vi "Main.vi"(10 "Sub Panel":refnum<vi>, 11 "Module Admin":refnum<class "Delacor_lib_QMH_Module Admin.lvclass">) -> ()   [LabVIEW 2019, in "Save DB_SQLite.lvlib"]
doc: "This template is based off of the Queued Message Handler design pattern and the Queued Message Handler project template that ships with LabVIEW.\n\nThe main difference is that the queue is private to this module and communication between modules is performed via Broadcast and Request events.\n\nRequest events are wrapped in public API methods and are handled in the Event Handling Loop (EHL) of this VI. Any module can register for Broadcast events sent by this module. The EHL generates messages based on user interface actions.\n\nThe Message Handling Loop (MHL) processes messages generated by the EHL, or by other messages. The messages are string values, so new messages can be added easily to the Message Cases case structure in the MHL. Each message cluster can also provide an optional value for Message Data, which is a variant that can be converted to whatever message-specific data is required.\n_____\nBased on Delacor QMH Project Template 5.0.0.82."
uses:
  Save DB_SQLite.lvlib
  <vilib>/Delacor/Delacor QMH/Libraries/Module Admin_class/Delacor_lib_QMH_Module Admin.lvclass
  Module Data--cluster.ctl
  Stop helper loop Argument--cluster.ctl
  Stop Argument--cluster.ctl
  <vilib>/Delacor/Delacor QMH/Libraries/Message Queue_class/Delacor_lib_QMH_Message Queue.lvclass/Delacor_lib_QMH_Message Queue.ctl
  <vilib>/Delacor/Delacor QMH/Libraries/Module Admin_class/Delacor_lib_QMH_Module Admin.lvclass/Delacor_lib_QMH_Module Admin.ctl
  <vilib>/Utility/miscctls.llb/LVPointTypeDef.ctl
  <vilib>/drjdpowell/SQLite Library/SQL Connection/Open (path).vi
  <vilib>/Delacor/Delacor QMH/Libraries/Message Queue_class/Delacor_lib_QMH_Enqueue Message (Single).vi
  <vilib>/Delacor/Delacor QMH/Libraries/Module Admin_class/Delacor_lib_QMH_Get External Launch.vi
  <vilib>/drjdpowell/SQLite Library/SQL Connection/Open (string).vi
  <vilib>/AdvancedString/Path To Command Line String.vi
  <vilib>/drjdpowell/SQLite Library/SQL Connection/Execute SQL (No results).vi
  <vilib>/Utility/error.llb/Error Cluster From Error Code.vi
  <vilib>/drjdpowell/SQLite Library/SQL Connection/Connection.lvclass
  <vilib>/ErrorRing/Error Ring.xnode
  <vilib>/Delacor/Delacor QMH/Libraries/Message Queue_class/Delacor_lib_QMH_Message Queue.lvclass
  <vilib>/drjdpowell/SQLite Library/SQLite.lvlib
  Analisis/Analisis.lvlib
panel:
  out "error out":errorcluster
  out "Status":string
types:
  T1 = typedef "Save DB_SQLite.lvlib/Request Events--cluster.ctl" = cluster{"Stop Module":refnum<user-event>, "Show Panel":refnum<user-event>, "Hide Panel":refnum<user-event>, "Get Module Execution Status":refnum<user-event>, "Show Diagram":refnum<user-event>, "Start Helper Loop":refnum<user-event>, "Stop helper loop":refnum<user-event>, "Set Waveform":refnum<user-event>, "Save_Data_From_Analisis":refnum<user-event>}
  T2 = typedef "Save DB_SQLite.lvlib/Module Data--cluster.ctl" = cluster{"Status":string}
  T3 = typedef "Save DB_SQLite.lvlib/Stop helper loop Argument--cluster.ctl" = cluster{"Boolean":bool}
  T4 = enum32{"invalid lock state", "Not Locked", "Locked (No Password)", "Password-protected"}
  T5 = typedef "Save DB_SQLite.lvlib/Stop Argument--cluster.ctl" = cluster{"Origin":string, "Exit via Stop Module Req?":bool, "Wait for Module to stop?":bool}
  T6 = typedef "LVPointTypeDef.ctl" = cluster{"Horizontal":i16, "Vertical":i16}
  T7 = enum32{"Invalid", "Standard", "Closed", "Hidden", "Minimized", "Maximized"}
  T8 = cluster{"Humedad":dbl, "Temperatura":dbl, "Voltaje":dbl, "Corriente":dbl, "Resistencia":i32}
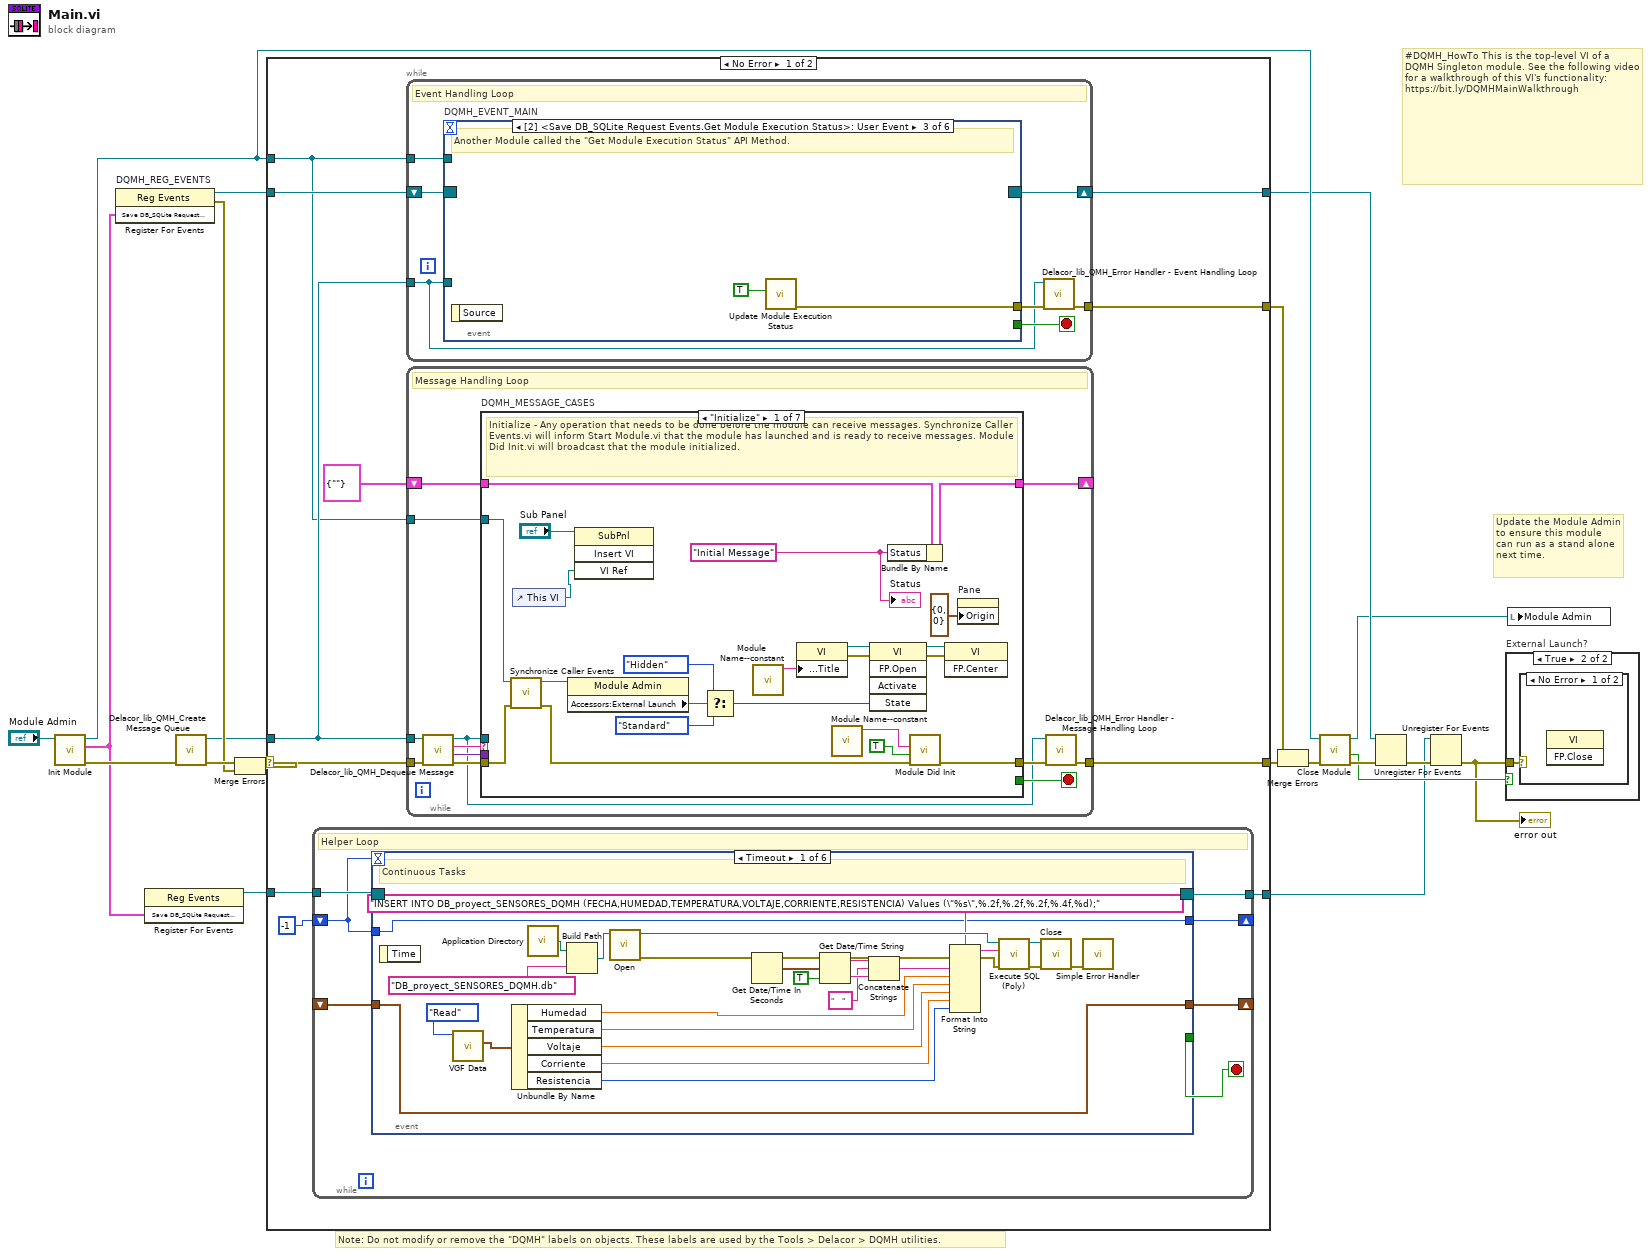
[diagram p0: block diagram]
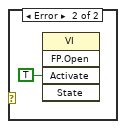
[diagram p3: hidden frame]
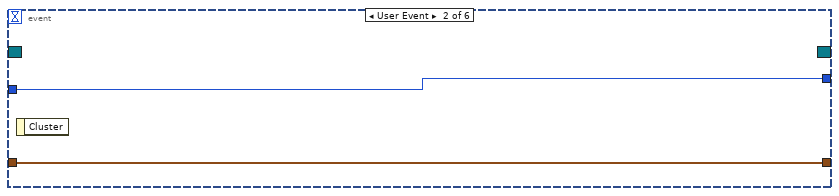
[diagram p4: hidden frame]
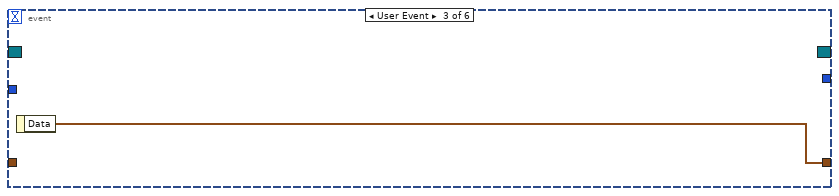
[diagram p5: hidden frame]
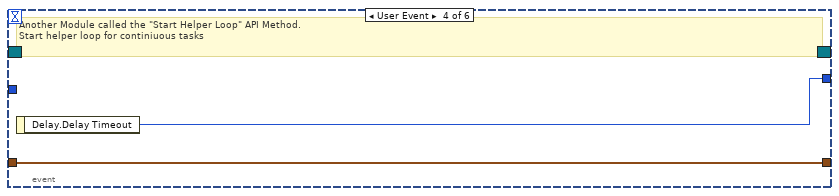
[diagram p6: hidden frame]
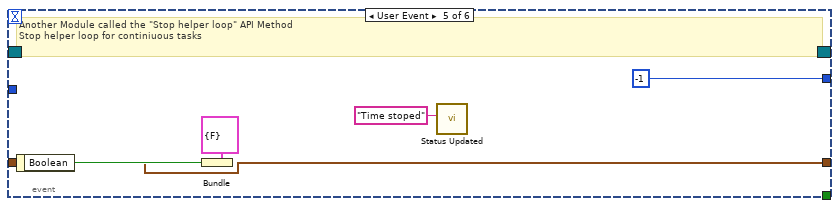
[diagram p7: hidden frame]
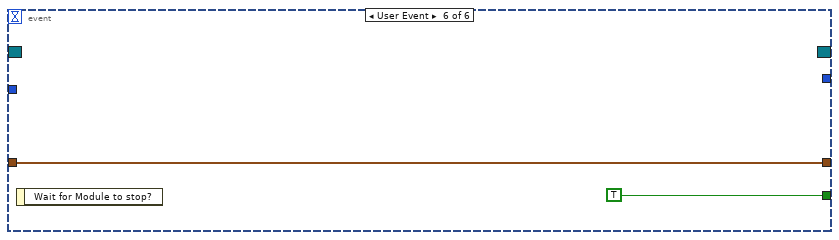
[diagram p8: hidden frame]
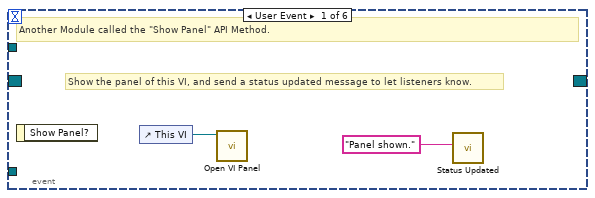
[diagram p9: hidden frame]
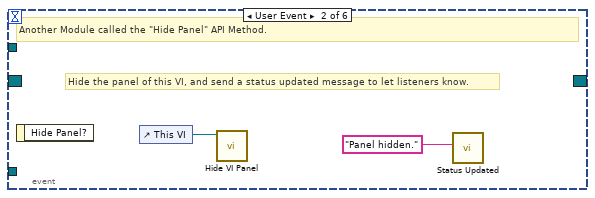
[diagram p10: hidden frame]
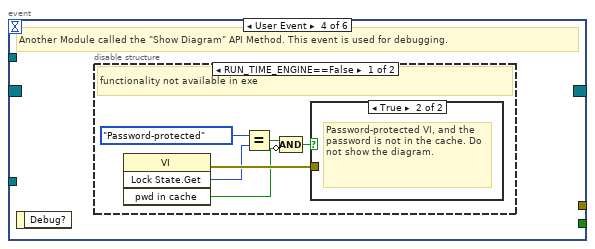
[diagram p11: hidden frame]
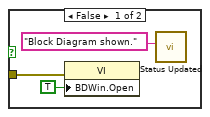
[diagram p12: hidden frame]
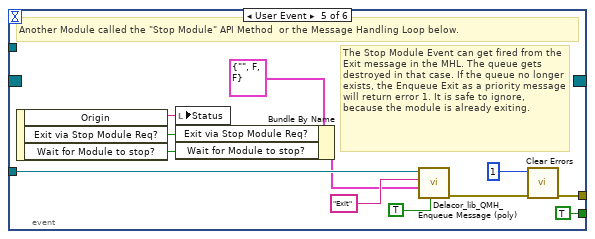
[diagram p14: hidden frame]
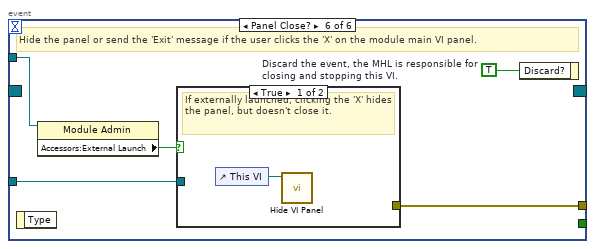
[diagram p15: hidden frame]
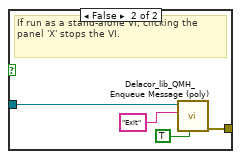
[diagram p16: hidden frame]
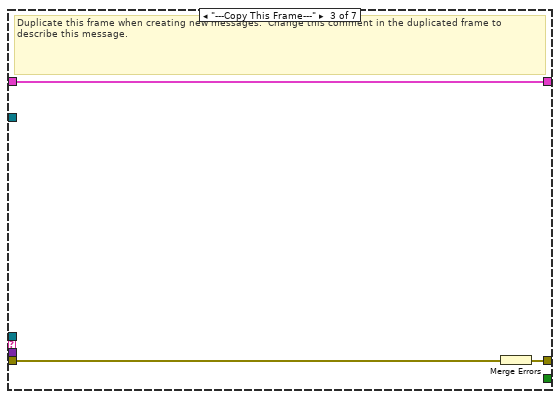
[diagram p18: hidden frame]
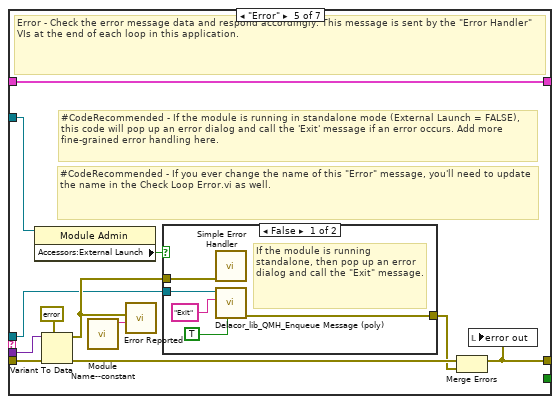
[diagram p20: hidden frame]
diagram:
  # "#DQMH_HowTo This is the top-level VI of a DQMH Singleton module. See the following video for a walkthrough of this VI's functionality: https://bit.ly/DQMHMainWalkthrough"
  # "Note: Do not modify or remove the \"DQMH\" labels on objects. These labels are used by the Tools > Delacor > DQMH utilities."
  # "Update the Module Admin to ensure this module can run as a stand alone next time."
  n1 = call "Init Module.vi"("Singleton Module Admin in"="Module Admin") -> ("error out"=w19:errorcluster, "Save DB_SQLite Request Events"=w4:T1, "Singleton Module Admin out"=w12:refnum<class "Delacor_lib_QMH_Module Admin.lvclass">)  [unwired: 8 in]
  n2 = register-events "DQMH_REG_EVENTS"(w4) -> (reference out=w10:refnum<event-registration>, error out=w13:errorcluster)  [unwired: 2 in]
  n3 = register-events(w4) -> (reference out=w5:refnum<event-registration>)  [unwired: 2 in, 1 out]
  n4 = call <vilib>:"Delacor_lib_QMH_Create Message Queue.vi"("error in (no error)"=w19) -> ("error out"=w15:errorcluster, "Message Queue"=w9:refnum<class "Delacor_lib_QMH_Message Queue.lvclass">)  [unwired: 9 in]
  n5 = Merge Errors(w15, w13) -> (w14:errorcluster)
  n6 = case shown="No Error" w14 {
    selector: w14 -> [w29 w209]
    tunnel: [w31 w208] -> w20
    tunnel: [w28 w214] -> w11
    tunnel: w10 -> [w26 w214]
    tunnel: w9 -> [w25 w207]
    tunnel: [w30 _] -> w17
    tunnel: w12 -> [w24 w210]
    tunnel: w5 -> [w23 _]
    tunnel: [w22 _] -> w1
    frame No Error {
      n7 = while {
        tunnel: w23 -> [w38]
        tunnel: [w37] -> w22
        shift-right: [w36] -> _
        shift-left: -1 -> [w32]
        shift-right: [w34] -> _
        shift-left: _ -> [w33]
        stop <- w35 stop-if-true
        # "Helper Loop"
        n8 = event shown="[0] Timeout" {
          selector: w38 -> [_ _ _ _ _ _]
          dyn-events: [_ _ _ _ _ _] -> w37
          timeout: w32 -> [_ _ _ _ _ _]
          tunnel: [w41 w65 _ w68 -1 _] -> w36
          tunnel: w32 -> [w41 w65 _ _ _ _]
          tunnel: [_ _ _ _ _ TRUE] -> w35
          tunnel: [w63 w64 w66 w67 w69 w74] -> w34
          tunnel: w33 -> [w63 w64 _ w67 w69 w74]
          event Timeout {
            # "Continuous Tasks"
            n9 = event-data() -> ()  [unwired: 1 in, 1 out]
            n10 = call "VGF Data.vi"("Accion"=enum16{"Read", "Set_data"}."Read") -> ("Data 2"=w39:T8)  [unwired: 10 in]
            n11 = Unbundle By Name(w39) -> ("Humedad"=w46:dbl, "Temperatura"=w45:dbl, "Voltaje"=w44:dbl, "Corriente"=w43:dbl, "Resistencia"=w42:i32)
            n12 = call <vilib>:"Application Directory.vi"() -> ("Application Directory"=w57:path)
            n13 = Build Path(base path=w57, name or relative path="DB_proyect_SENSORES_DQMH.db") -> (appended path=w55:path)
            n14 = call-poly <vilib>:"Open.vi"("db file"=w55) -> ("error out"=w59:errorcluster, "SQLite Connection"=w62:refnum<class "Connection.lvclass">)  [unwired: 9 in]
            n15 = Get Date/Time In Seconds() -> (seconds since 1Jan1904=w52:timestamp)
            n16 = Get Date/Time String(seconds (now)=w52, want seconds? (F)=TRUE) -> (date string=w50:string, time string=w48:string)  [unwired: 1 in]
            n17 = Concatenate Strings(w50, "    " ("string"), w48) -> (w49:string)
            n18 = Format Into String(format string="INSERT INTO DB_proyect_SENSORES_DQMH (FECHA,HUMEDAD,TEMPERATURA,VOLTAJE,CORRIENTE,RESISTENCIA) Values (\"%s\",%.2f,%.2f,%.2f,%.4f,%d);", w49, w46, w45, w44, w43, w42) -> (resulting string=w54:string)  [unwired: 2 in, 1 out]
            n19 = call-poly <vilib>:"Execute SQL (Poly).vi"("error in (no error)"=w59, "SQL"=w54, "SQLite Connection in"=w62) -> ("error out"=w60:errorcluster, "SQLite Connection"=w61:refnum<class "Connection.lvclass">)  [unwired: 7 in]
            n20 = call-dynamic "Close.vi"("error in (no error)"=w60, "SQLite Connection in"=w61) -> ("error out"=w58:errorcluster)  [unwired: 9 in]
            n21 = call <vilib>:"Simple Error Handler.vi"("error in (no error)"=w58) -> ()  [unwired: 4 in, 5 out]
          }
          event User Event {
            n22 = event-data() -> ()  [unwired: 1 in, 1 out]
          }
          event User Event {
            n23 = event-data() -> ("Data"=w66:T8)  [unwired: 1 in]
          }
          event User Event {
            # "Another Module called the \"Start Helper Loop\" API Method.\nStart helper loop for continiuous tasks"
            n24 = event-data() -> ("Delay.Delay Timeout"=w68:i32)  [unwired: 1 in]
          }
          event User Event {
            # "Another Module called the \"Stop helper loop\" API Method\nStop helper loop for continiuous tasks"
            n25 = event-data() -> ("Boolean"=w72:bool)  [unwired: 1 in]
            n26 = Bundle(cluster=T3 {"Boolean"=FALSE} ("Stop helper loop Argument"), "Boolean"=w72) -> ()  [unwired: 1 out]
            n27 = call "Status Updated.vi"("Status"="Time stoped") -> ()  [unwired: 10 in, 1 out]
          }
          event User Event {
            n28 = event-data() -> ()  [unwired: 1 in, 1 out]
          }
        }
      }
      n29 = while {
        tunnel: w25 -> [w76]
        shift-right: [w79] -> w28
        shift-left: w26 -> [w80]
        tunnel: [w81] -> w30
        tunnel: w24 -> [w77]
        stop <- w78 stop-if-true
        # "Event Handling Loop"
        n30 = event "DQMH_EVENT_MAIN" shown="[2] <Save DB_SQLite Request Events.Get Module Execution Status>: User Event" {
          selector: w80 -> [_ _ _ _ _ _]
          dyn-events: [_ _ _ _ _ _] -> w79
          timeout: _ -> [_ _ _ _ _ _]
          tunnel: [_ _ _ _ TRUE ("Discard?") _] -> w78
          tunnel: w76 -> [_ _ _ _ w105 w112]
          tunnel: [_ _ w88 _ w108 w114] -> w82
          tunnel: w77 -> [_ _ _ _ _ w111]
          event User Event {
            # "Show the panel of this VI, and send a status updated message to let listeners know."
            # "Another Module called the \"Show Panel\" API Method."
            n31 = event-data() -> ()  [unwired: 1 in, 1 out]
            n32 = control-ref of="This VI"() -> (w84:refnum<vi>)
            n33 = call "Open VI Panel.vi"("VI"=w84) -> ()  [unwired: 10 in, 1 out]
            n34 = call "Status Updated.vi"("Status"="Panel shown." ("format string")) -> ()  [unwired: 10 in, 1 out]
          }
          event User Event {
            # "Hide the panel of this VI, and send a status updated message to let listeners know."
            # "Another Module called the \"Hide Panel\" API Method."
            n35 = event-data() -> ()  [unwired: 1 in, 1 out]
            n36 = control-ref of="This VI"() -> (w86:refnum<vi>)
            n37 = call "Hide VI Panel.vi"("VI"=w86) -> ()  [unwired: 10 in, 1 out]
            n38 = call "Status Updated.vi"("Status"="Panel hidden." ("format string")) -> ()  [unwired: 10 in, 1 out]
          }
          event User Event {
            # "Another Module called the \"Get Module Execution Status\" API Method."
            n39 = event-data() -> ()  [unwired: 1 in, 1 out]
            n40 = call "Update Module Execution Status.vi"("Running?"=TRUE) -> ("error out"=w88:errorcluster)  [unwired: 10 in]
          }
          event User Event {
            # "Another Module called the \"Show Diagram\" API Method. This event is used for debugging."
            n41 = event-data() -> ()  [unwired: 1 in, 1 out]
            n42 = disable-structure shown="RUN_TIME_ENGINE==False" {
              frame condition #0 (active) {
                # "functionality not available in exe"
                n43 = invoke class="VI" method="Lock State.Get"() -> (error out=w94:errorcluster, "Get Lock State"=w93:T4, "pwd in cache"=w90:bool)  [unwired: 4 in, 1 out]
                n44 = Equal?(x=T4."Password-protected", y=w93) -> (x = y?=w91:bool)
                n45 = Compound Arithmetic op=AND(w91, invert w90) -> (w89:bool)
                n46 = case shown="True" w89 {
                  tunnel: w94 -> [w97 _]
                  frame False {
                    n47 = property class="VI"(error in=w97, "BDWin.Open"=TRUE ("Block Diagram Window:Open")) -> ()  [unwired: 1 in, 2 out]
                    n48 = call "Status Updated.vi"("Status"="Block Diagram shown." ("format string")) -> ()  [unwired: 10 in, 1 out]
                  }
                  frame True {
                    # "Password-protected VI, and the password is not in the cache. Do not show the diagram."
                  }
                }
              }
              frame condition #1 {
              }
            }
          }
          event User Event {
            # "The Stop Module Event can get fired from the Exit message in the MHL. The queue gets destroyed in that case. If the queue no longer exists, the Enqueue Exit as a priority message will return error 1. It is safe to ignore, because the module is already exiting."
            # "Another Module called the \"Stop Module\" API Method  or the Message Handling Loop below."
            n49 = event-data() -> ("Origin"=w104:string, "Exit via Stop Module Req?"=w100:bool, "Wait for Module to stop?"=w99:bool)  [unwired: 1 in]
            n50 = local write "Status"(w104) -> ()
            n51 = Bundle By Name(cluster=T5 {"Origin"="", "Exit via Stop Module Req?"=FALSE, "Wait for Module to stop?"=FALSE} ("Stop Argument"), "Exit via Stop Module Req?"=w100, "Wait for Module to stop?"=w99) -> (w98:T5)
            n52 = call-poly <vilib>:"Delacor_lib_QMH_Enqueue Message (poly).vi"("Priority Message? (F)"=TRUE, "Message Data"=w98, "Message"="Exit", "Message Queue in"=w105) -> ("error out"=w109:errorcluster)  [unwired: 6 in, 1 out]
            n53 = call <vilib>:"Clear Errors.vi"("error in (no error)"=w109, "specific error code to clear (0: all)"=1) -> ("error out"=w108:errorcluster)  [unwired: 4 in, 1 out]
          }
          event Panel Close? {
            w113 = TRUE  # Discard the event, the MHL is responsible for closing and stopping this VI.
            # "Hide the panel or send the 'Exit' message if the user clicks the 'X' on the module main VI panel."
            n54 = event-data() -> ()  [unwired: 1 in, 1 out]
            n55 = property class="Module Admin"(reference=w111) -> ("Accessors:External Launch"=w110:bool)  [unwired: 1 in, 2 out]
            n56 = case shown="True" w110 {
              tunnel: w112 -> [_ w118]
              tunnel: [_ w119] -> w114
              frame True {
                # "If externally launched, clicking the 'X' hides the panel, but doesn't close it."
                n57 = control-ref of="This VI"() -> (w115:refnum<vi>)
                n58 = call "Hide VI Panel.vi"("VI"=w115) -> ()  [unwired: 10 in, 1 out]
              }
              frame False {
                # "If run as a stand-alone VI, clicking the panel 'X' stops the VI."
                n59 = call-poly <vilib>:"Delacor_lib_QMH_Enqueue Message (poly).vi"("Priority Message? (F)"=TRUE, "Message"="Exit", "Message Queue in"=w118) -> ("error out"=w119:errorcluster)  [unwired: 7 in, 1 out]
              }
            }
            n60 = event-data("Discard?"=w113) -> ()  [unwired: 1 in, 1 out]
          }
        }
        n61 = call-dynamic "Delacor_lib_QMH_Error Handler - Event Handling Loop.vi"("error in (no error)"=w82, "Message Queue in"=w76) -> ("dup error in"=w81:errorcluster)  [unwired: 8 in, 1 out]
      }
      n62 = while {
        tunnel: w25 -> [w122]
        shift-right: [w126] -> _
        shift-left: T2 {"Status"=""} ("Data Cluster") -> [w127]
        tunnel: w29 -> [w130]
        tunnel: [w128] -> w31
        tunnel: w24 -> [w120]
        stop <- w125 stop-if-true
        # "Message Handling Loop"
        n63 = call-dynamic "Delacor_lib_QMH_Dequeue Message.vi"("error in (no error)"=w130, "Message Queue in"=w122) -> ("error out"=w129:errorcluster, "Message Data"=w123:variant, "Message"=w124:string, "Message Queue out"=w121:refnum<class "Delacor_lib_QMH_Message Queue.lvclass">)  [unwired: 6 in]
        n64 = case "DQMH_MESSAGE_CASES" shown="\"Initialize\"" w124 {
          selector: w124 -> [_ _ _ _ _ _ w194]
          tunnel: w121 -> [_ _ _ _ w164 w186 _]
          tunnel: w129 -> [w151 w155 w158 w160 w171 w192 w196]
          tunnel: [w149 w155 w157 w160 w167 w189 w197] -> w131
          tunnel: w127 -> [w140 w154 w156 w159 w166 w185 w195]
          tunnel: [w139 w154 w156 w159 w166 w185 w195] -> w126
          tunnel: [_ _ _ _ _ w184 _] -> w125
          tunnel: w123 -> [_ _ _ _ w165 w183 _]
          tunnel: w120 -> [w141 _ _ _ w163 w178 _]
          frame "Initialize" {
            w134 = "Initial Message" ("Initial Message")
            # "Initialize - Any operation that needs to be done before the module can receive messages. Synchronize Caller Events.vi will inform Start Module.vi that the module has launched and is ready to receive messages. Module Did Init.vi will broadcast that the module initialized."
            n65 = call "Synchronize Caller Events.vi"("error in (no error)"=w151, "Singleton Module Admin in"=w141) -> ("error out"=w150:errorcluster, "Singleton Module Admin out"=w136:refnum<class "Delacor_lib_QMH_Module Admin.lvclass">)  [unwired: 8 in]
            n66 = control-ref of="This VI"() -> (w132:refnum<vi>)
            n67 = property class="Module Admin"(reference=w136) -> ("Accessors:External Launch"=w145:bool)  [unwired: 1 in, 2 out]
            n68 = invoke class="SubPnl" method="Insert VI"(reference="Sub Panel", "VI Ref"=w132) -> ()  [unwired: 2 in, 4 out]
            n69 = Select(t=T7."Hidden" ("State"), s=w145, f=T7."Standard" ("State")) -> (s? t:f=w142:T7)
            n70 = call "Module Name--constant.vi"() -> ("Module Name"=w148:string)  [unwired: 11 in]
            n71 = property class="VI"("Front Panel.Title"=w148) -> (reference out=w147:refnum<vi>, error out=w153:errorcluster)  [unwired: 2 in]
            n72 = call "Module Name--constant.vi"() -> ("Module Name"=w137:string)  [unwired: 11 in]
            n73 = invoke class="VI" method="FP.Open"(reference=w147, error in=w153, "State"=w142) -> (reference out=w146:refnum<vi>, error out=w152:errorcluster)  [unwired: 2 in, 3 out]
            n74 = Bundle By Name(cluster=w140, "Status"=w134) -> (w139:T2)
            n75 = call "Module Did Init.vi"("error in (no error)"=w150, "Initialized?"=TRUE, "Origin"=w137) -> ("error out"=w149:errorcluster)  [unwired: 8 in]
            n76 = invoke class="VI" method="FP.Center"(reference=w146, error in=w152) -> ()  [unwired: 1 in, 3 out]
            n77 = property on="Pane" class="Pane"("Origin"=T6 {"Horizontal"=0, "Vertical"=0}) -> ()  [unwired: 2 in, 2 out]
            "Status" <- w134
          }
          frame "--- Module Specific ---" {
            # "Separator -- The following cases handle messages specific to this Module."
          }
          frame "---Copy This Frame---" {
            # "Duplicate this frame when creating new messages.  Change this comment in the duplicated frame to describe this message."
            n78 = Merge Errors(w158) -> (w157:errorcluster)
          }
          frame "--- Exit and Error Handling---" {
            # "Separator - The following cases handle errors and exit messages."
          }
          frame "Error" {
            # "#CodeRecommended - If you ever change the name of this \"Error\" message, you'll need to update the name in the Check Loop Error.vi as well."
            # "#CodeRecommended - If the module is running in standalone mode (External Launch = FALSE), this code will pop up an error dialog and call the 'Exit' message if an error occurs. Add more fine-grained error handling here."
            # "Error - Check the error message data and respond accordingly. This message is sent by the \"Error Handler\" VIs at the end of each loop in this application."
            n79 = property class="Module Admin"(reference=w163) -> ("Accessors:External Launch"=w162:bool)  [unwired: 1 in, 2 out]
            n80 = Variant To Data(error in=w171, type=errorcluster {"status"=FALSE, "code"=0, "source"=""} ("error constant"), Variant=w165) -> (data=w172:errorcluster, error out=w169:errorcluster)
            n81 = call "Module Name--constant.vi"() -> ("Module Name"=w161:string)  [unwired: 11 in]
            n82 = call "Error Reported.vi"("Additional Information"=w161, "Error"=w172) -> ()  [unwired: 9 in, 1 out]
            n83 = case shown="False" w162 {
              tunnel: [w177 _] -> w168
              tunnel: w164 -> [w175 _]
              tunnel: w172 -> [w176 _]
              frame False {
                # "If the module is running standalone, then pop up an error dialog and call the \"Exit\" message."
                n84 = call <vilib>:"Simple Error Handler.vi"("error in (no error)"=w176) -> ()  [unwired: 4 in, 5 out]
                n85 = call-poly <vilib>:"Delacor_lib_QMH_Enqueue Message (poly).vi"("Priority Message? (F)"=TRUE, "Message"="Exit", "Message Queue in"=w175) -> ("error out"=w177:errorcluster)  [unwired: 7 in, 1 out]
              }
              frame True {
                # "If the module was launched externally, calling the Error Reported broadcast VI is the only action performed by the \"Error\" message. The module's caller can then process the error appropriately."
              }
            }
            n86 = Merge Errors(w169, w168) -> (w167:errorcluster)
            n87 = local write "error out"(w167) -> ()
          }
          frame "Exit" {
            w182 = 91  # 91: not all Exit messages will have an argument
            w184 = TRUE  # Stop the VI
            # "Release the message queue reference"
            # "#CodeNeeded - Add any required cleanup code here"
            # "Exit - Exit the application."
            n88 = Variant To Data(error in=w192, type=T5 {"Origin"="", "Exit via Stop Module Req?"=FALSE, "Wait for Module to stop?"=FALSE} ("Stop Argument"), Variant=w183) -> (data=w180:T5, error out=w188:errorcluster)
            n89 = call <vilib>:"Clear Errors.vi"("error in (no error)"=w188, "specific error code to clear (0: all)"=w182) -> ("error out"=w191:errorcluster)  [unwired: 4 in, 1 out]
            n90 = control-ref of="This VI"() -> (w179:refnum<vi>)
            n91 = call-dynamic "Delacor_lib_QMH_Release Message Queue.vi"("error in (no error)"=w191, "Message Queue"=w186) -> ("error out"=w190:errorcluster)  [unwired: 9 in]
            n92 = call "Handle Exit.vi"("Stop Argument"=w180, "Admin in"=w178, "VI reference"=w179) -> ("error out"=w187:errorcluster)  [unwired: 7 in, 1 out]
            n93 = Merge Errors(w190, w187) -> (w189:errorcluster)
          }
          frame Default {
            # "'Default' case only runs if there is a message that isn't defined in any of the other cases.  Output a programming error."
            n94 = call "Module Name--constant.vi"() -> ("Module Name"=w193:string)  [unwired: 11 in]
            n95 = xnode "Error Ring"("parameter 0"=w194, "parameter 1"=w193) -> ("error out"=w198:errorcluster)
            n96 = Merge Errors(w196, w198) -> (w197:errorcluster)
          }
        }
        n97 = call-dynamic "Delacor_lib_QMH_Error Handler - Message Handling Loop.vi"("error in (no error)"=w131, "Message Queue in"=w121) -> ("dup error in"=w128:errorcluster)  [unwired: 8 in, 1 out]
      }
    }
    frame Error {
      # "Synchronize Caller Events.vi will inform Start Module.vi that the module has launched and will let the code calling Start Module.vi register for broadcasts and would permit the caller receive the broadcast that an error occurred at launch time."
      n98 = call-dynamic "Delacor_lib_QMH_Release Message Queue.vi"("error in (no error)"=w209, "Message Queue"=w207) -> ("error out"=w208:errorcluster)  [unwired: 9 in]
      n99 = call "Synchronize Caller Events.vi"("Singleton Module Admin in"=w210) -> ("error out"=w215:errorcluster)  [unwired: 9 in, 1 out]
      n100 = call "Module Name--constant.vi"() -> ("Module Name"=w213:string)  [unwired: 11 in]
      n101 = Format Into String(format string="An error occurred during initialization. %s is no longer running.", w213) -> (resulting string=w211:string)  [unwired: 2 in, 1 out]
      n102 = Merge Errors(w208, w215) -> (w216:errorcluster)
      n103 = call "Error Reported.vi"("Additional Information"=w211, "Error"=w216) -> ()  [unwired: 9 in, 1 out]
    }
  }
  n104 = Merge Errors(w17, w20) -> (w16:errorcluster)
  n105 = call "Close Module.vi"("error in (no error)"=w16, "Module Admin in"=w12) -> ("error out"=w18:errorcluster, "External Launch"=w6:bool, "Module Admin out"=w7:refnum<class "Delacor_lib_QMH_Module Admin.lvclass">)  [unwired: 7 in]
  n106 = Unregister For Events(event registration refnum=w11, error in=w18) -> (error out=w3:errorcluster)
  n107 = Unregister For Events(event registration refnum=w1, error in=w3) -> (error out=w2:errorcluster)
  "error out" <- w2
  n108 = case "External Launch?" shown="True" w6 {
    tunnel: w2 -> [_ w217]
    frame False {
    }
    frame True {
      n109 = case shown="No Error" w217 {
        frame No Error {
          n110 = invoke class="VI" method="FP.Close"() -> ()  [unwired: 3 in, 3 out]
        }
        frame Error {
          n111 = invoke class="VI" method="FP.Open"("Activate"=TRUE ("Activate?")) -> ()  [unwired: 4 in, 5 out]
        }
      }
    }
  }
  n112 = local write "Module Admin"(w7) -> ()
